vi "checkYield95.vi"() -> ()   [LabVIEW 2012]
uses:
  <vilib>/addons/database/Auxilliary.llb/DB Tools Cursor Type.ctl
  <vilib>/addons/database/Connection.llb/DB Tools Open Connec (Path).vi
  <vilib>/addons/database/Connection.llb/Conn Execute.vi
  <vilib>/addons/database/Recordset.llb/Rec Fetch Recordset Data (R).vi
  <vilib>/addons/database/Recordset.llb/Rec Destroy - Connection.vi
  <vilib>/addons/database/Recordset.llb/Rec Fetch Double Data (R).vi
  <vilib>/addons/database/_DB Variant To Data/Database Variant To Data.xnode
  <vilib>/addons/database/NI_Database_API.lvlib
panel:
  out "error out 2":errorcluster
  out "Boolean":bool
  out "result":i16
  out "Numeric":i32
  out "spreadsheet string":string
  out "concatenated string":string
  out "array":string[][](array[string])
  out "error out":errorcluster
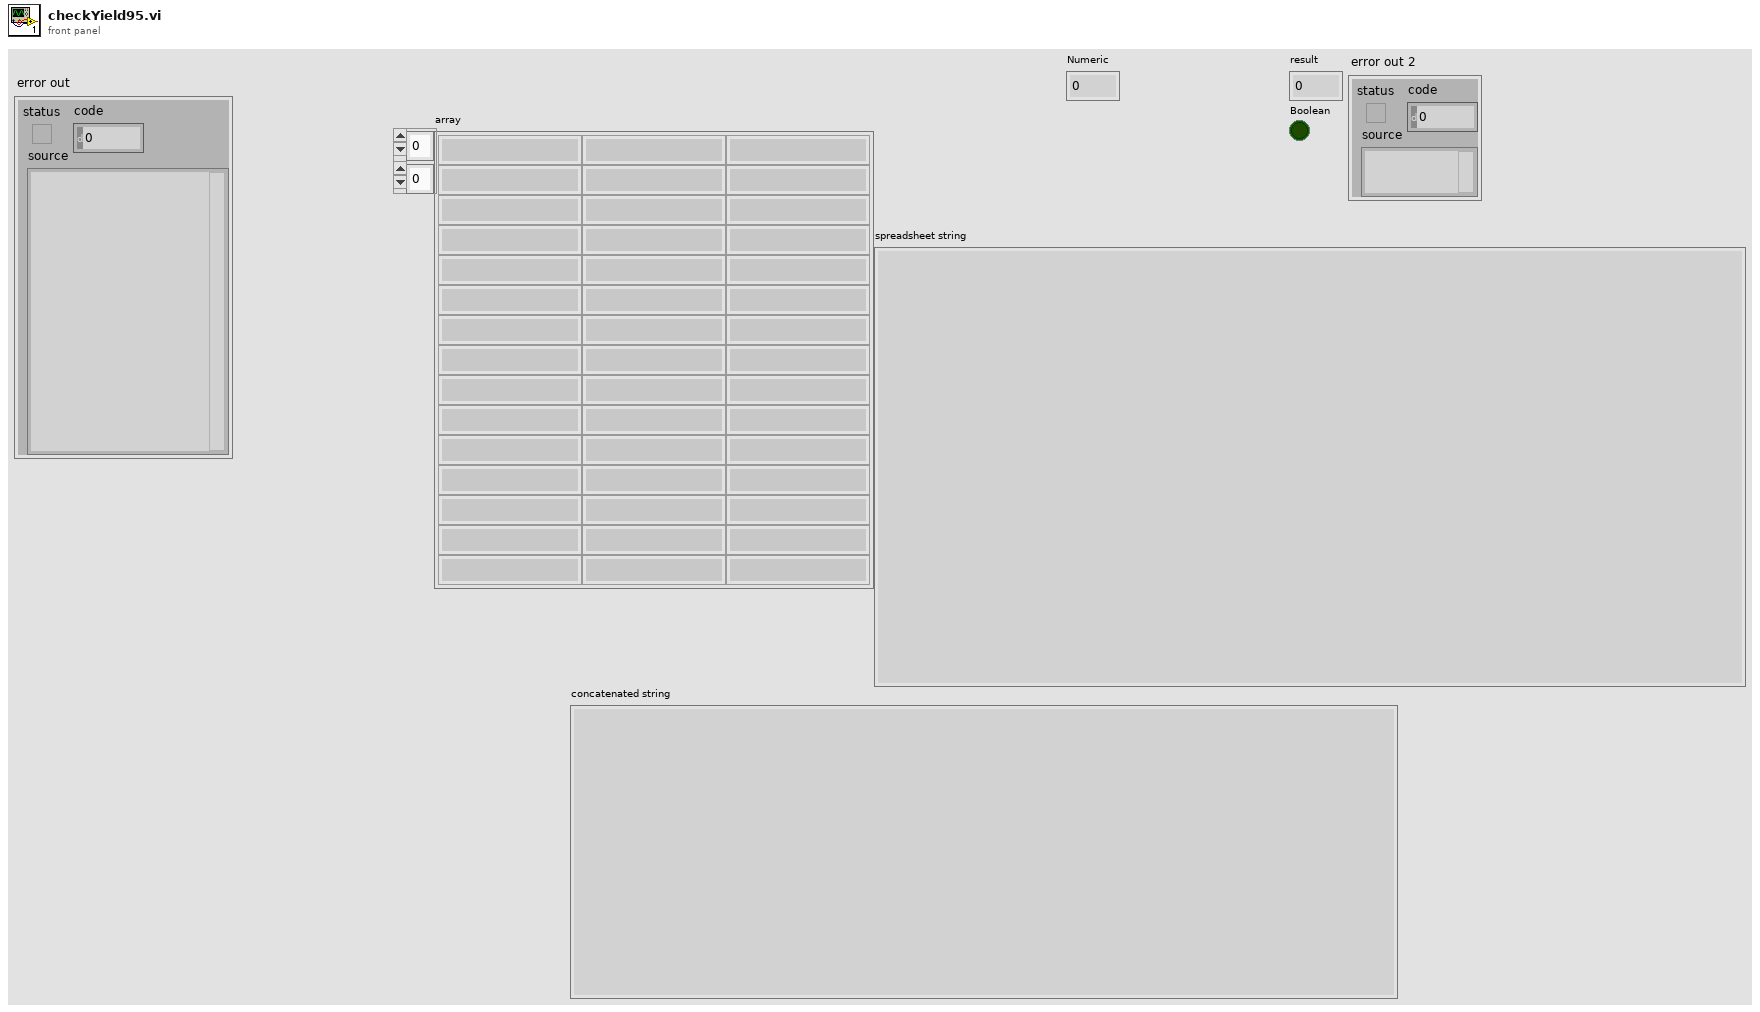
[diagram p1: front panel]
types:
  T1 = typedef "NI_Database_API.lvlib/DB Tools Cursor Type.ctl" = enum16{"forward-only", "keyset", "dynamic", "static"}
  T2 = typedef "NI_Database_API.lvlib/Conn ObjectReference.ctl" = refnum<k1>
  T3 = typedef "NI_Database_API.lvlib/Rec ObjectReference.ctl" = refnum<k1>
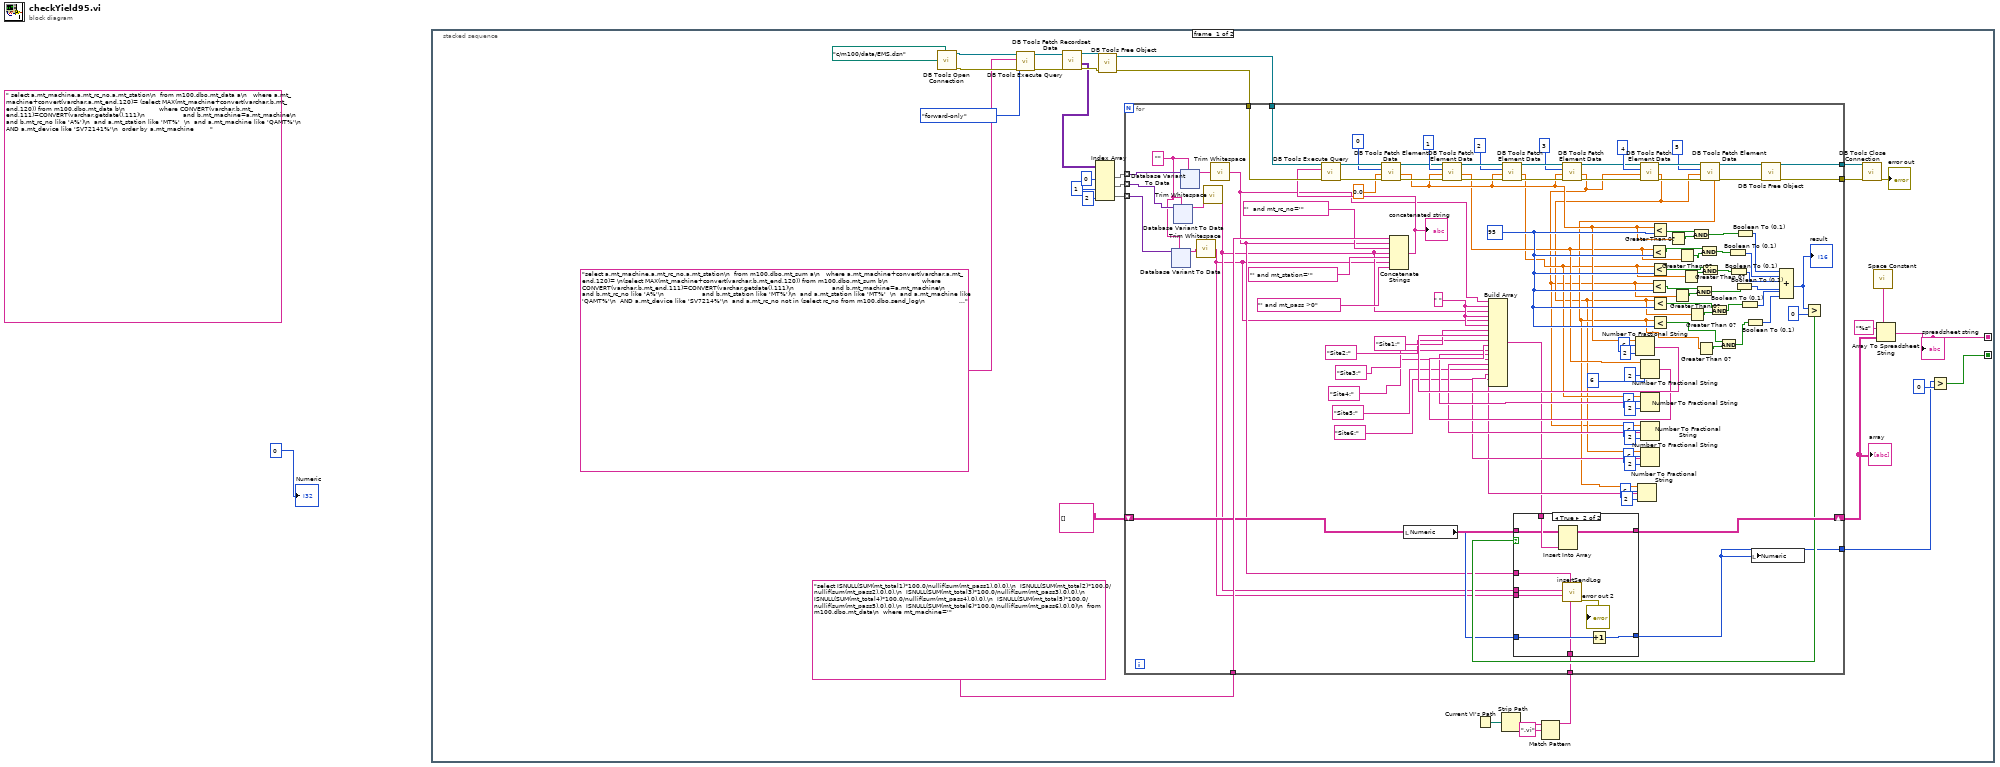
[diagram p0: block diagram]
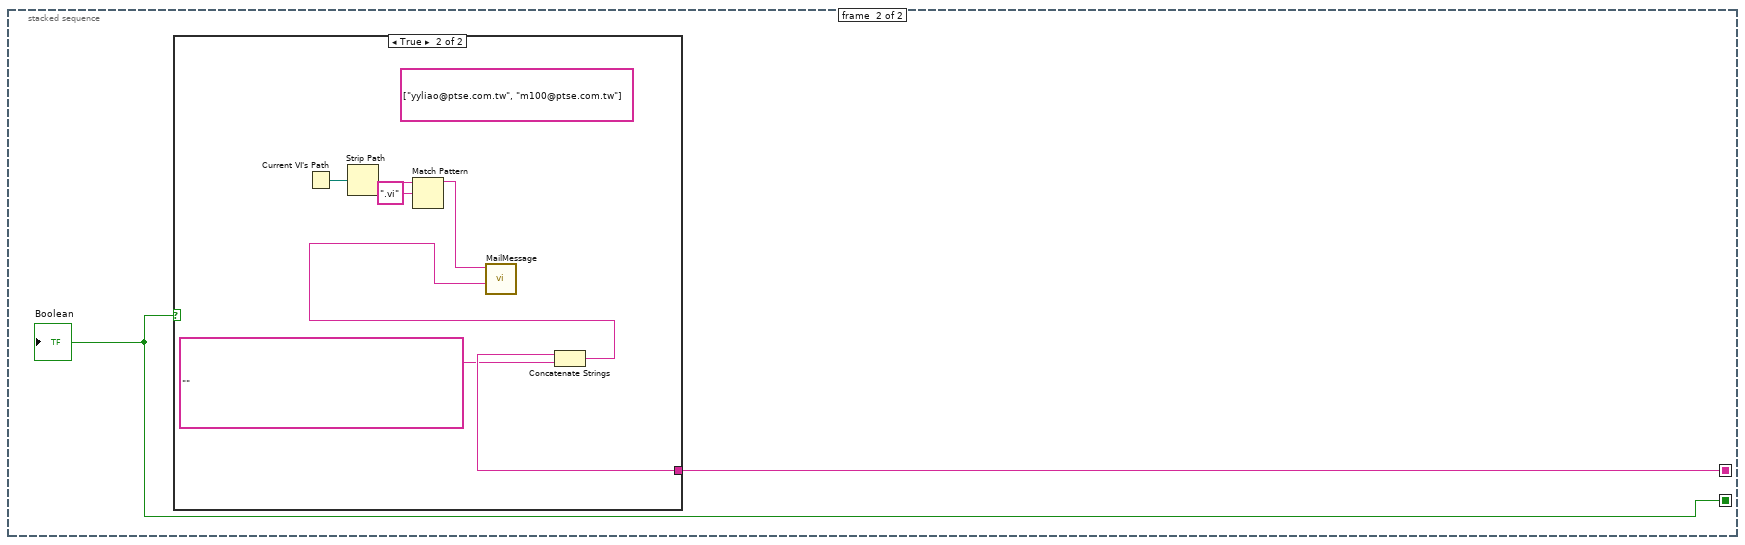
[diagram p3: hidden frame]
diagram:
  (unwired) " select a.mt_machine,a.mt_rc_no,a.mt_station\n  from m100.dbo.mt_data a\n   where a.mt_machine+convert(varchar,a.mt_end,120)= (select MAX(mt_machine+convert(varchar,b.mt_end,120)) from m100.dbo.mt_data b\n                 where CONVERT(varchar,b.mt_end,111)=CONVERT(varchar,getdate(),111)\n                   and b.mt_machine=a.mt_machine\n                   and b.mt_rc_no like 'A%')\n  and a.mt_station like 'MT%'  \n  and a.mt_machine like 'QAMT%'\n  AND a.mt_device like 'SV72141%'\n  order by a.mt_machine        "
  n1 = stacked-sequence {
    seq-local: [w23 _] -> [_ w250]
    seq-local: [w8 _] -> [_ w249]
    frame #0 {
      n2 = call-poly <vilib>:"DB Tools Open Connection.vi"("connection information"=path "c:/m100/data/EMS.dsn") -> ("error out"=w20:errorcluster, "connection reference"=w21:T2)  [unwired: 7 in]
      n3 = call-poly <vilib>:"DB Tools Execute Query.vi"("error in (no error)"=w20, "cursor type"=DB_Tools_Cursor_Type."forward-only", "SQL query"="select a.mt_machine,a.mt_rc_no,a.mt_station\n  from m100.dbo.mt_sum a\n   where a.mt_machine+convert(varchar,a.mt_end,120)= \n(select MAX(mt_machine+convert(varchar,b.mt_end,120)) from m100.dbo.mt_sum b\n                 where CONVERT(varchar,b.mt_end,111)=CONVERT(varchar,getdate(),111)\n                   and b.mt_machine=a.mt_machine\n                   and b.mt_rc_no like 'A%'\n                   and b.mt_station like 'MT%')\n  and a.mt_station like 'MT%'  \n  and a.mt_machine like 'QAMT%'\n  AND a.mt_device like 'SV7214%'\n  and a.mt_rc_no not in (select rc_no from m100.dbo.send_log\n                                             where program='checkYield95' \n                                                  and machine=a.mt_machine\n                                                  and step = a.mt_station)\n  order by a.mt_machine        ", "connection reference"=w21) -> ("error out"=w33:errorcluster, "recordset reference"=w34:T3)  [unwired: 4 in]
      n4 = call-poly <vilib>:"DB Tools Fetch Recordset Data.vi"("error in (no error)"=w33, "recordset reference"=w34) -> ("error out"=w31:errorcluster, "recordset data"=w19:variant[][], "recordset reference out"=w32:T3)  [unwired: 3 in]
      n5 = Index Array(array=w19, index (col) #1=0 ("disabled index (col)"), index (col) #2=1 ("index (col)"), index (col) #3=2 ("index (col)")) -> (element #1=w26:variant[], element #2=w25:variant[], element #3=w17:variant[])  [unwired: 3 in]
      n6 = call-poly <vilib>:"DB Tools Free Object.vi"("error in (no error)"=w31, "recordset reference"=w32) -> ("error out"=w15:errorcluster, "connection reference"=w16:T2)  [unwired: 8 in]
      n7 = Current VI's Path() -> (path=w5:path)
      n8 = Strip Path(path=w5) -> (name=w4:string)  [unwired: 1 out]
      n9 = Match Pattern(string=w4, regular expression=".vi") -> (before substring=w2:string)  [unwired: 1 in, 3 out]
      n10 = for {
        tunnel: w26 -> [w140] mode=indexing
        tunnel: w25 -> [w139] mode=indexing
        tunnel: w17 -> [w136] mode=indexing
        tunnel: w16 -> [w134]
        tunnel: w15 -> [w133]
        tunnel: "select ISNULL(SUM(mt_total1)*100.0/nullif(sum(mt_pass1),0),0),\n  ISNULL(SUM(mt_total2)*100.0/nullif(sum(mt_pass2),0),0),\n  ISNULL(SUM(mt_total3)*100.0/nullif(sum(mt_pass3),0),0),\n  ISNULL(SUM(mt_total4)*100.0/nullif(sum(mt_pass4),0),0),\n  ISNULL(SUM(mt_total5)*100.0/nullif(sum(mt_pass5),0),0),\n  ISNULL(SUM(mt_total6)*100.0/nullif(sum(mt_pass6),0),0)\n  from m100.dbo.mt_data\n  where mt_machine='" ("string") -> [w132]
        tunnel: [w110] -> w13
        tunnel: [w109] -> w12
        shift-right: [w72] -> w10
        shift-left: string[][] [] ("array") -> [w71]
        tunnel: [w40] -> w7
        tunnel: w2 -> [w36]
        w98 = " " ("element")
        w106 = 95 ("y")
        w135 = ""
        n11 = xnode "Database Variant To Data"("database variant"=w136, "type"=w135) -> ("data"=w67:string)  [unwired: 1 in, 1 out]
        n12 = xnode "Database Variant To Data"("database variant"=w139, "type"=w135) -> ("data"=w68:string)  [unwired: 1 in, 1 out]
        n13 = xnode "Database Variant To Data"("database variant"=w140, "type"=w135) -> ("data"=w69:string)  [unwired: 1 in, 1 out]
        n14 = call <vilib>:"Trim Whitespace.vi"("string"=w67) -> ("trimmed string"=w37:string)  [unwired: 1 in]
        n15 = call <vilib>:"Trim Whitespace.vi"("string"=w68) -> ("trimmed string"=w38:string)  [unwired: 1 in]
        n16 = call <vilib>:"Trim Whitespace.vi"("string"=w69) -> ("trimmed string"=w39:string)  [unwired: 1 in]
        n17 = Concatenate Strings(w132, w39, "'  and mt_rc_no='" ("string"), w38, "' and mt_station='" ("string"), w37, "' and mt_pass >0" ("string")) -> (w128:string)
        "concatenated string" <- w128
        n18 = call-poly <vilib>:"DB Tools Execute Query.vi"("error in (no error)"=w133, "SQL query"=w128, "connection reference"=w134) -> ("error out"=w137:errorcluster, "recordset reference"=w138:T3)  [unwired: 5 in]
        n19 = call-poly <vilib>:"DB Tools Fetch Element Data.vi"("error in (no error)"=w137, "type"=0.0, "column index"=0, "recordset reference"=w138) -> ("error out"=w116:errorcluster, "data"=w66:dbl, "recordset reference out"=w117:T3)  [unwired: 3 in]
        n20 = local read "Numeric"() -> (w41:i32)
        n21 = call-poly <vilib>:"DB Tools Fetch Element Data.vi"("error in (no error)"=w116, "type"=w66, "column index"=1, "recordset reference"=w117) -> ("error out"=w123:errorcluster, "data"=w58:dbl, "recordset reference out"=w127:T3)  [unwired: 3 in]
        n22 = call-poly <vilib>:"DB Tools Fetch Element Data.vi"("error in (no error)"=w123, "type"=w66, "column index"=2, "recordset reference"=w127) -> ("error out"=w122:errorcluster, "data"=w55:dbl, "recordset reference out"=w126:T3)  [unwired: 3 in]
        n23 = call-poly <vilib>:"DB Tools Fetch Element Data.vi"("error in (no error)"=w122, "type"=w66, "column index"=3, "recordset reference"=w126) -> ("error out"=w121:errorcluster, "data"=w42:dbl, "recordset reference out"=w111:T3)  [unwired: 3 in]
        n24 = Number To Fractional String(number=w66, width (-)=i16 6, precision (6)=i16 2) -> (F-format string=w96:string)  [unwired: 1 in]
        n25 = call-poly <vilib>:"DB Tools Fetch Element Data.vi"("error in (no error)"=w121, "type"=w42, "column index"=4, "recordset reference"=w111) -> ("error out"=w107:errorcluster, "data"=w47:dbl, "recordset reference out"=w125:T3)  [unwired: 3 in]
        n26 = Number To Fractional String(number=w58, width (-)=i16 6, precision (6)=i16 2) -> (F-format string=w82:string)  [unwired: 1 in]
        n27 = Number To Fractional String(number=w55, width (-)=i16 6, precision (6)=i16 2) -> (F-format string=w80:string)  [unwired: 1 in]
        n28 = Number To Fractional String(number=w42, width (-)=i16 6, precision (6)=i16 2) -> (F-format string=w79:string)  [unwired: 1 in]
        n29 = Number To Fractional String(number=w47, width (-)=i16 6, precision (6)=i16 2) -> (F-format string=w77:string)  [unwired: 1 in]
        n30 = Less?(x=w58, y=w106) -> (x < y?=w60:bool)
        n31 = Less?(x=w42, y=w106) -> (x < y?=w43:bool)
        n32 = Less?(x=w66, y=w106) -> (x < y?=w63:bool)
        n33 = Less?(x=w55, y=w106) -> (x < y?=w54:bool)
        n34 = Less?(x=w47, y=w106) -> (x < y?=w46:bool)
        n35 = Greater Than 0?(x=w66) -> (x > 0?=w64:bool)
        n36 = Greater Than 0?(x=w42) -> (x > 0?=w45:bool)
        n37 = Greater Than 0?(x=w58) -> (x > 0?=w61:bool)
        n38 = Greater Than 0?(x=w55) -> (x > 0?=w57:bool)
        n39 = Greater Than 0?(x=w47) -> (x > 0?=w49:bool)
        n40 = And(x=w63, y=w64) -> (x .and. y?=w62:bool)
        n41 = And(x=w43, y=w45) -> (x .and. y?=w44:bool)
        n42 = And(x=w60, y=w61) -> (x .and. y?=w59:bool)
        n43 = call-poly <vilib>:"DB Tools Fetch Element Data.vi"("error in (no error)"=w107, "type"=w47, "column index"=5, "recordset reference"=w125) -> ("error out"=w120:errorcluster, "data"=w50:dbl, "recordset reference out"=w124:T3)  [unwired: 3 in]
        n44 = Number To Fractional String(number=w50, width (-)=i16 6, precision (6)=i16 2) -> (F-format string=w74:string)  [unwired: 1 in]
        n45 = Build Array(w39, w98, w38, w98, w37, w98, "Site1:" ("element"), w96, "Site2:" ("element"), w82, "Site3:" ("element"), w80, "Site4:" ("element"), w79, "Site5:" ("element"), w77, "Site6:" ("element"), w74) -> (w73:string[])
        n46 = Less?(x=w50, y=w106) -> (x < y?=w51:bool)
        n47 = Greater Than 0?(x=w50) -> (x > 0?=w53:bool)
        n48 = And(x=w54, y=w57) -> (x .and. y?=w56:bool)
        n49 = And(x=w46, y=w49) -> (x .and. y?=w48:bool)
        n50 = And(x=w51, y=w53) -> (x .and. y?=w52:bool)
        n51 = Boolean To (0,1)(Boolean=w59) -> (0, 1=w105:i16)
        n52 = Boolean To (0,1)(Boolean=w56) -> (0, 1=w104:i16)
        n53 = Boolean To (0,1)(Boolean=w44) -> (0, 1=w103:i16)
        n54 = Boolean To (0,1)(Boolean=w62) -> (0, 1=w65:i16)
        n55 = Boolean To (0,1)(Boolean=w48) -> (0, 1=w102:i16)
        n56 = Boolean To (0,1)(Boolean=w52) -> (0, 1=w101:i16)
        n57 = call-poly <vilib>:"DB Tools Free Object.vi"("error in (no error)"=w120, "recordset reference"=w124) -> ("error out"=w109:errorcluster, "connection reference"=w110:T2)  [unwired: 8 in]
        n58 = Compound Arithmetic op=ADD(w65, w105, w104, w103, w102, w101) -> (w100:i16)
        "result" <- w100
        n59 = Greater?(x=w100, y=i16 0) -> (0:w70:bool)
        n60 = case shown="True" w70 {
          tunnel: w73 -> [_ w152]
          tunnel: [w142 w151] -> w72
          tunnel: w71 -> [w142 w150]
          tunnel: [w141 w149] -> w40
          tunnel: w41 -> [w141 w148]
          tunnel: w39 -> [_ w147]
          tunnel: w38 -> [_ w146]
          tunnel: w37 -> [_ w145]
          tunnel: w36 -> [_ w144]
          frame False {
          }
          frame True {
            n61 = Insert Into Array(array=w150, new element=w152) -> (w151:string[][])  [unwired: 2 in]
            n62 = call "insertSendLog.vi"("Program"=w144, "Machine"=w147, "step"=w145, "rc_no"=w146) -> ("error out"=→"error out 2":errorcluster)  [unwired: 7 in]
            n63 = Increment(x=w148) -> (x+1=w149:i32)
          }
        }
        n64 = local write "Numeric"(w40) -> ()
      }
      "array" <- w10
      n65 = call <vilib>:"DB Tools Close Connection.vi"("error in (no error)"=w12, "connection reference"=w13) -> ("error out"=→"error out":errorcluster)  [unwired: 5 in]
      n66 = call <vilib>:"Space Constant.vi"() -> ("String"=w22:string)
      n67 = Array To Spreadsheet String(delimiter (Tab)=w22, array=w10, 3:"%s" ("format string")) -> (spreadsheet string=w23:string)
      "spreadsheet string" <- w23
      n68 = Greater?(x=w7, y=0) -> (0:w8:bool)
    }
    frame #1 {
      n69 = case shown="True" w249 {
        tunnel: w250 -> [_ w257]
        frame False {
        }
        frame True {
          (unwired) string[] ["yyliao@ptse.com.tw", "m100@ptse.com.tw"] ("recipients")
          n70 = Current VI's Path() -> (path=w255:path)
          n71 = Strip Path(path=w255) -> (name=w254:string)  [unwired: 1 out]
          n72 = Match Pattern(string=w254, regular expression=".vi") -> (before substring=w252:string)  [unwired: 1 in, 3 out]
          n73 = Concatenate Strings(w257, "" ("string")) -> (w251:string)
          n74 = call "MailMessage.vi"("message"=w251, "program"=w252) -> ()  [unwired: 10 in]
        }
      }
      "Boolean" <- w249
    }
  }
  "Numeric" <- 0 ("Numeric")
